vi "LC2_Comm_main.vi"() -> ()   [LabVIEW 2016]
uses:
  <vilib>/DNP3/DNP3_Master/Operation Mode.ctl
  <vilib>/DNP3/DNP3_Master/Poll Binary Input Variation.ctl
  <vilib>/DNP3/DNP3_Master/Analog Variation.ctl
  <vilib>/DNP3/DNP3_Master/Poll Analog Input Variation.ctl
  <vilib>/DNP3/DNP3_Master/Response Type.ctl
  <vilib>/DNP3/DNP3_Master/Start Stop.ctl
  <vilib>/DNP3/DNP3_Master/Analog Info.ctl
  BESS_LC/LC_BESS_global.vi
  Communication/Global communication.vi
  Communication/Global communication output.vi
  Communication/DNP3 communication files/MGCC Communication Files/DNP3_Master_Station_MGCC.lvlib
  <vilib>/DNP3/DNP3_Master.lvlib
panel:
  out "Startup time":dbl
  out "Array":T3(array[cluster])=[{"DNP3 channel"="Master/Channel 160.36.56.207: 18000", "DNP3 master"="Master", "DNP3 master session"="Master/Channel 160.36.56.207: 18000/Master Session 9-10", "DNP3 command"="Master/Channel 160.36.56.207: 18000/Master Session 9-10/Command ", "MS_Network_Settings_Initial"={"Outstation IP"="160.36.56.207", "DNP3 Port"=18000, "DNP3 Master Address"=9, "DNP3 Outstation Address"=10}, "Ping status"=enum."Success", "PollD"=[{"start"=0, "stop"=5}], "PollA"=[{"start"=0, "stop"=5}], "error out"={"status"=FALSE, "code"=5103, "source"="DNP3_Master_Station_MGCC.lvlib:LC1_MS_Main.vi:580001<ERR>\nCommunication timeout\n\n\n<b>Complete call chain:</b>\n     DNP3_Master_Station_MGCC.lvlib:LC1_MS_Main.vi:580001\n     LC2_Comm_main.vi"}, "MS_RESET_IND"=FALSE}]
  out "BESS LC communication":dbl[](array[numeric])=[0.0, 1.0369910801229782, 77.34308905073745, 0.0, 0.0, 0.5]
  out "OS SubVI Iterations":i16=6647
  in  "RESET OS":bool caption="Reset Outstation"
  in  "ENABLE OS":bool=TRUE
  out "OS SETTINGS CHANGED":bool
  out "MS POLLING? IND":bool=TRUE
  in  "Settings Cluster":T4={"Default Variation:Analog Input Event (OBJ32)"=1, "Default Variation:Analog Input (OBJ30)"=1, "Default Variation:Binary Input (OBJ01)"=1, "Default Variation:Analog Output (OBJ40)"=4, "Default Variation:Binary Output Event (OBJ11)"=1, "Default Variation:Binary Output (OBJ10)"=1, "Default Variation:Analog Output Event (OBJ42)"=8, "Unsolicited Response Allowed"=FALSE, "Control:Select Timeout (ms)"=0, "Misc:Appl Confirmation Timeout"=0} {"Default Variation:Analog Output Event (OBJ42)" items=["32-bit without Time"=1, "16-bit without Time"=2, "32-bit with Time"=3, "16-bit with Time"=4, "Single-prec without Time"=5, "Double-prec without Time"=6, "Single-prec with Time"=7, "Double-prec with Time"=8]; "Default Variation:Binary Output (OBJ10)" items=["Packed Format"=1, "Output Status with Flags"=2]; "Default Variation:Binary Output Event (OBJ11)" items=["Status without Time"=1, "Status with Time"=2]; "Default Variation:Analog Output (OBJ40)" items=["32-bit with Flag"=1, "16-bit with Flag"=2, "Single-prec with Flag"=3, "Double-prec with Flag"=4]; "Default Variation:Binary Input (OBJ01)" items=["Packed Format"=1, "With Flags"=2]; "Default Variation:Analog Input (OBJ30)" items=["32-bit with Flag"=1, "16-bit with Flag"=2, "32-bit without Flag"=3, "16-bit without Flag"=4, "Single-prec with Flag"=5, "Double-prec with Flag"=6]; "Default Variation:Analog Input Event (OBJ32)" items=["32-bit without Time"=1, "16-bit without Time"=2, "32-bit with Time"=3, "16-bit with Time"=4, "Single-prec without Time"=5, "Double-prec without Time"=6, "Single-prec with Time"=7, "Double-prec with Time"=8]}
  in  "Network Settings 1":T5={"port (20000)"=18000, "Master IP"="10.38.59.110", "Master Address"=12340, "Outstation Address "=54320, " update rate"=50}
  in  "DNP3 DataMap 1":T6={"Binary Output Points"=1, "Binary Input Points"=0, "Analog Output Points"=22, "Analog Input Points"=22}
  out "Numeric 3":i32
  out "LC1_MS_TX_Status_Binary":T1=enum."Cancel"
  out "LC1_MS_TX_Status_Analog":T1=enum."Success"
  out "LC1_MS_RX_Status_Binary":T1=enum."Cancel"
  out "LC1_MS_RX_Status_Analog":T1=enum."Success"
  out "Analog Input":dbl[](array[numeric])=[0.0, 1.0369911365960325, 77.34322413077294, 0.0, 0.0, 0.5]
  in  "LC1_MS_Network_Settings":T7={"Outstation IP"="160.36.56.207", "DNP3 Port"=18000, "DNP3 Master Address"=9, "DNP3 Outstation Address"=10}
  in  "Poll Enable":T8={"En_Rx_An"=TRUE, "En_Tx_An"=TRUE, "En_Rx_Di"=FALSE, "En_Tx_Di"=FALSE}
  in  "ENABLE MS":bool=TRUE
  in  "RESET MS":bool caption="Reset Outstation"
  in  "LC1_MS_DNP3_Settings":T13={"Binary Out Mode"=6, "Binary In Variation"=0, "Analog Out Variation"=4, "Analog Out Mode"=6, "Analog In Variation"=6} {"Analog In Variation" items=["Default", "32-bit with Flag", "16-bit with Flag", "32-bit without Flag", "16-bit without Flag", "Single-prec with Flag", "Double-prec with Flag"]; "Analog Out Mode" items=["SBO"=0, "Select"=3, "Operate"=4, "Direct"=5, "Direct No Ack"=6]; "Analog Out Variation" items=["32-bit"=1, "16-bit"=2, "Single-prec"=3, "Double-prec"=4]; "Binary In Variation" items=["Default", "Packed Format", "With Flags"]; "Binary Out Mode" items=["SBO"=0, "Select"=3, "Operate"=4, "Direct"=5, "Direct No Ack"=6]}
  out "Numeric":i32=3331
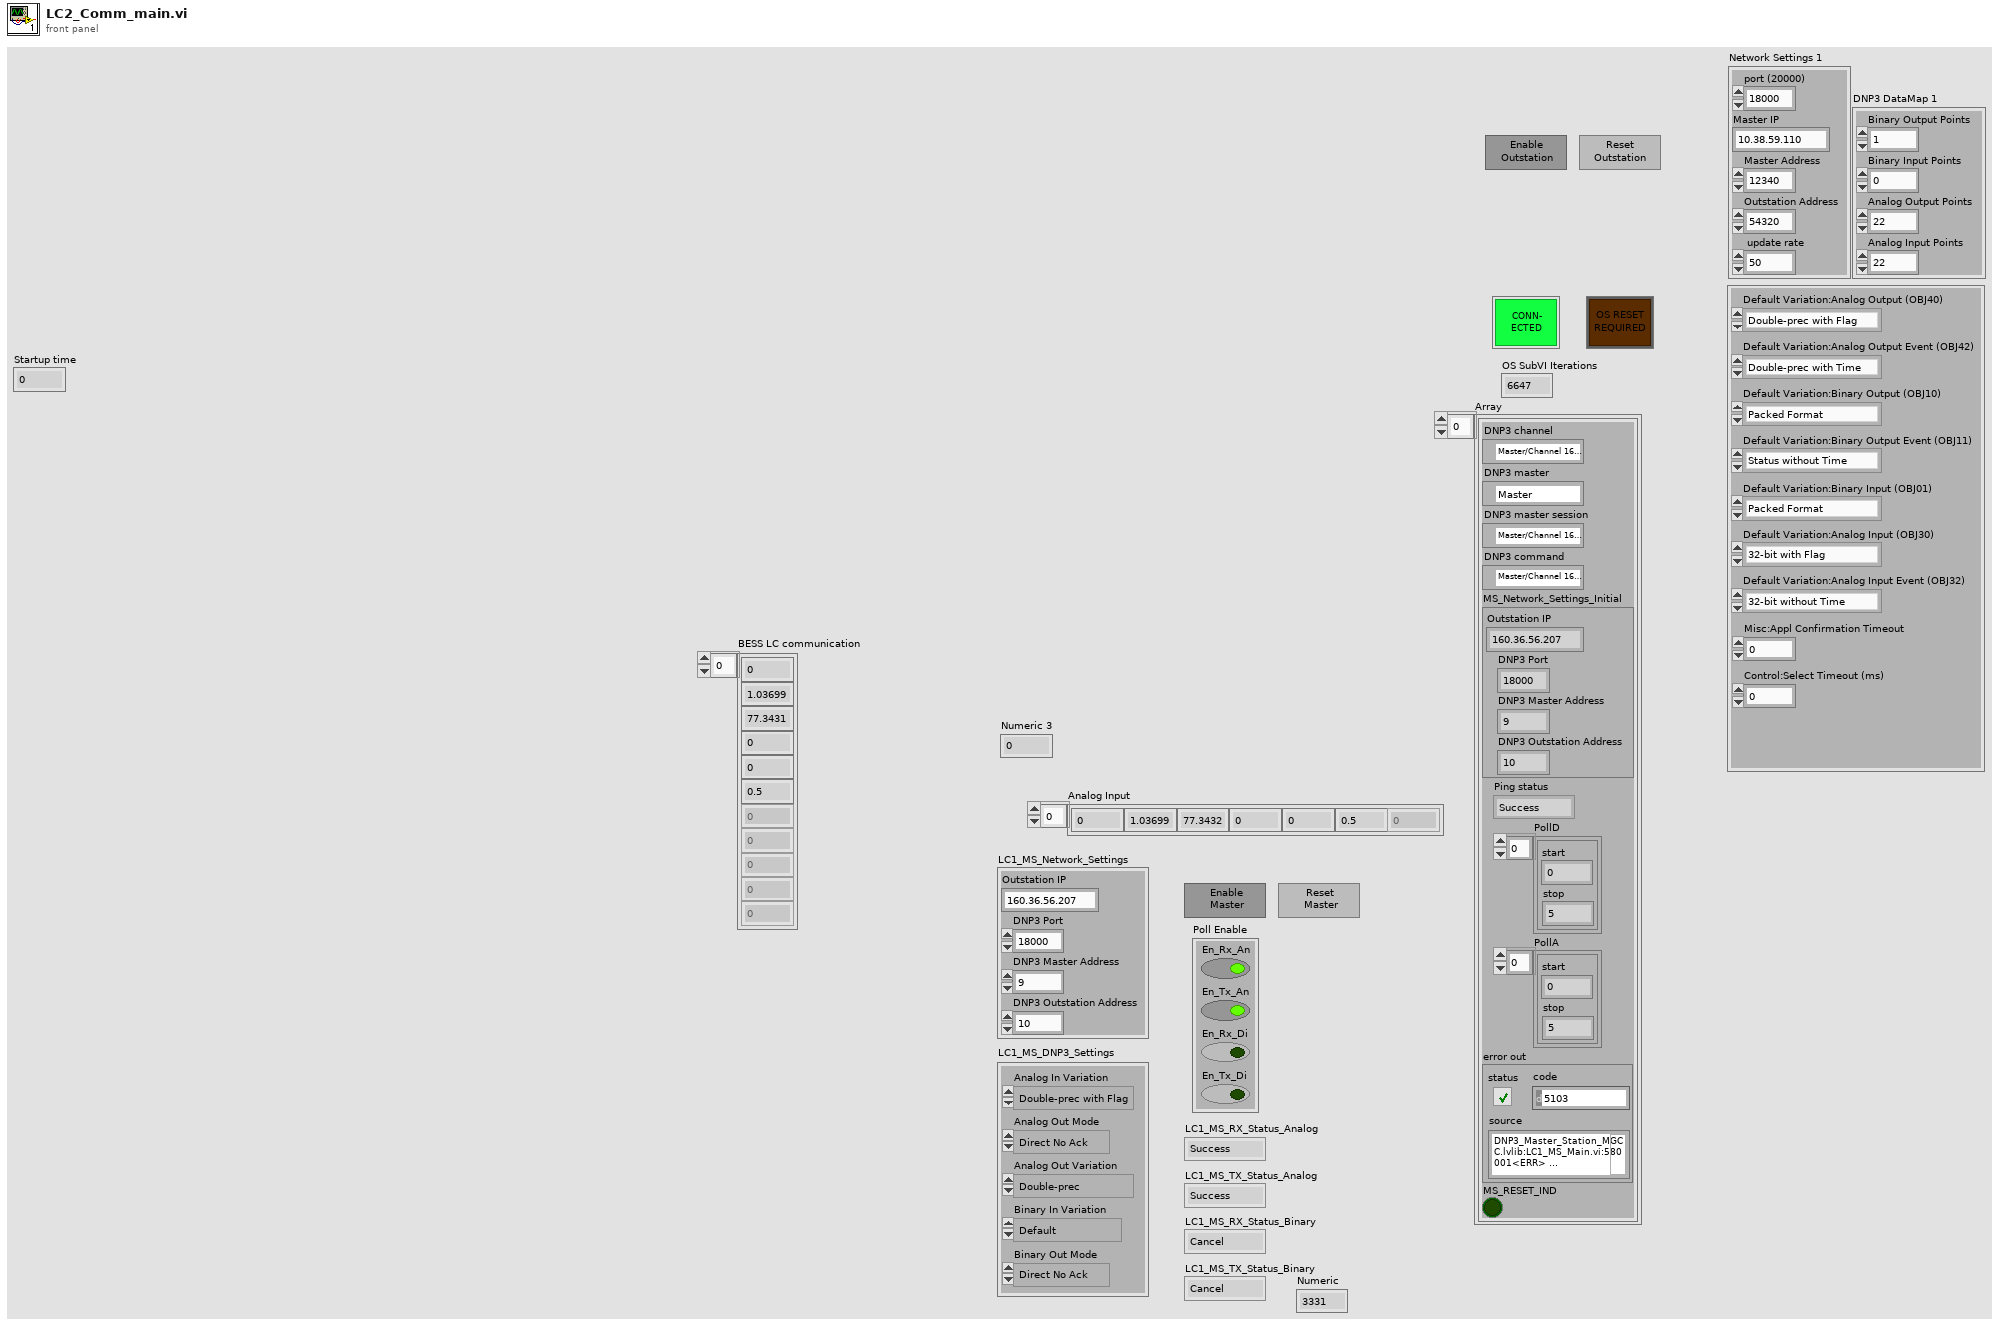
[diagram p1: front panel]
types:
  T1 = typedef "DNP3_Master.lvlib/Response Type.ctl" = enum16{"Idle", "Buffering", "Pending", "Success", "Failure", "Mismatch", "Status Code", "IIN", "Timeout", "Cancel"}
  T2 = typedef "DNP3_Master.lvlib/Start Stop.ctl" = cluster{"start":u16, "stop":u16}
  T3 = cluster{"DNP3 channel":refnum<k21>, "DNP3 master":refnum<k21>, "DNP3 master session":refnum<k21>, "DNP3 command":refnum<k21>, "MS_Network_Settings_Initial":cluster{"Outstation IP":string, "DNP3 Port":u16, "DNP3 Master Address":u16, "DNP3 Outstation Address":u16}, "Ping status":T1, "PollD":T2[], "PollA":T2[], "error out":errorcluster, "MS_RESET_IND":bool}[]
  T4 = cluster{"Default Variation:Analog Input Event (OBJ32)":u8, "Default Variation:Analog Input (OBJ30)":u8, "Default Variation:Binary Input (OBJ01)":u8, "Default Variation:Analog Output (OBJ40)":u8, "Default Variation:Binary Output Event (OBJ11)":u8, "Default Variation:Binary Output (OBJ10)":u8, "Default Variation:Analog Output Event (OBJ42)":u8, "Unsolicited Response Allowed":bool, "Control:Select Timeout (ms)":u32, "Misc:Appl Confirmation Timeout":u32}
  T5 = cluster{"port (20000)":u16, "Master IP":string, "Master Address":u16, "Outstation Address ":u16, " update rate":u32}
  T6 = cluster{"Binary Output Points":u16, "Binary Input Points":u16, "Analog Output Points":u16, "Analog Input Points":u16}
  T7 = cluster{"Outstation IP":string, "DNP3 Port":u16, "DNP3 Master Address":u16, "DNP3 Outstation Address":u16}
  T8 = cluster{"En_Rx_An":bool, "En_Tx_An":bool, "En_Rx_Di":bool, "En_Tx_Di":bool}
  T9 = typedef "DNP3_Master.lvlib/Operation Mode.ctl" = u8
  T10 = typedef "DNP3_Master.lvlib/Poll Binary Input Variation.ctl" = u8
  T11 = typedef "DNP3_Master.lvlib/Analog Variation.ctl" = u8
  T12 = typedef "DNP3_Master.lvlib/Poll Analog Input Variation.ctl" = u8
  T13 = cluster{"Binary Out Mode":T9, "Binary In Variation":T10, "Analog Out Variation":T11, "Analog Out Mode":T9, "Analog In Variation":T12}
  T14 = typedef "DNP3_Master.lvlib/Analog Info.ctl" = cluster{"index":u16, "value":dbl}
  T15 = cluster{"Binary Out Mode":T9, "Binary In Variation":T10, "Analog Out Variation":T11, "Analog Out Mode":T9, "Analog In Variation":T12}[]
  T16 = cluster{"En_Rx_An":bool, "En_Tx_An":bool, "En_Rx_Di":bool, "En_Tx_Di":bool}[]
  T17 = cluster{"Outstation IP":string, "DNP3 Port":u16, "DNP3 Master Address":u16, "DNP3 Outstation Address":u16}[]
  T18 = cluster{"response status":T1, "response status":T1, "response status":T1, "response status":T1}
  T19 = cluster{"DNP3 channel":refnum<k21>, "DNP3 master":refnum<k21>, "DNP3 master session":refnum<k21>, "DNP3 command":refnum<k21>, "MS_Network_Settings_Initial":cluster{"Outstation IP":string, "DNP3 Port":u16, "DNP3 Master Address":u16, "DNP3 Outstation Address":u16}, "Ping status":T1, "PollD":T2[], "PollA":T2[], "error out":errorcluster, "MS_RESET_IND":bool}
  T20 = cluster{"DNP3 outstation session out":refnum<k21>, "DNP3 outstation out":refnum<k21>, "error out":errorcluster}
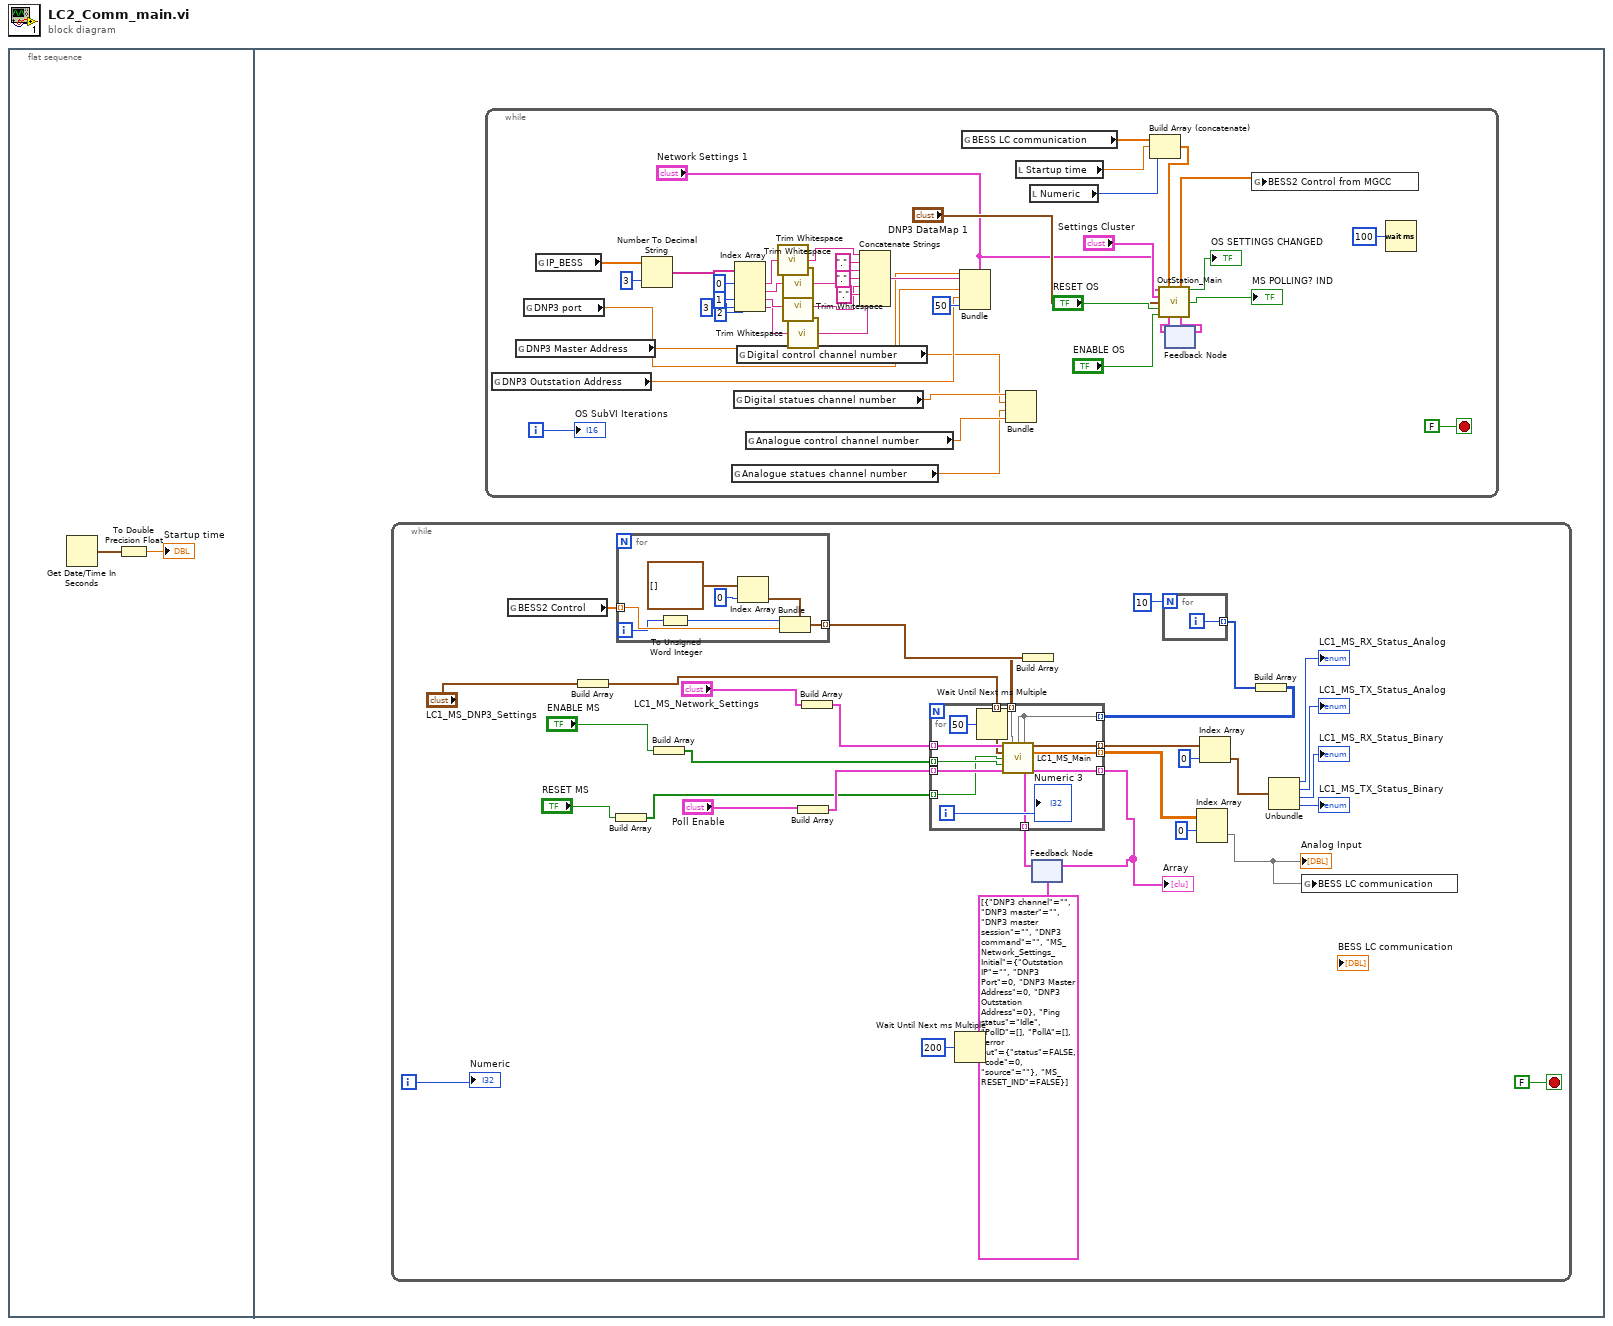
[diagram p0: block diagram]
diagram:
  n1 = flat-sequence {
    frame #0 {
      n2 = Get Date/Time In Seconds() -> (seconds since 1Jan1904=w2:timestamp)
      n3 = To Double Precision Float(number=w2) -> (double precision float=→"Startup time":dbl)
    }
    frame #1 {
      n4 = while {
        i -> [w9]
        stop <- FALSE stop-if-true
        n5 = global read "Global communication output.vi" "BESS2 Control"() -> (w13:dbl[])
        n6 = Build Array("LC1_MS_DNP3_Settings") -> (w14:T15)
        n7 = Build Array("RESET MS") -> (w16:bool[])
        n8 = for {
          tunnel: [w42] -> w12 mode=indexing
          tunnel: w13 -> [w37] mode=indexing
          i -> [w36]
          n9 = To Unsigned Word Integer(number=w36) -> (unsigned 16bit integer=w38:u16)
          n10 = Index Array(array=T14[] [] ("values"), index=0) -> (element=w39:T14)
          n11 = Bundle(cluster=w39, "index"=w38, "value"=w37) -> (w42:T14)
        }
        n12 = Build Array("ENABLE MS") -> (w18:bool[])
        n13 = Build Array("Poll Enable") -> (w20:T16)
        n14 = Build Array("LC1_MS_Network_Settings") -> (w22:T17)
        n15 = Wait Until Next ms Multiple(millisecond multiple=u32 200) -> ()  [unwired: 1 out]
        n16 = Build Array(w12) -> (w11:T14[][])
        n17 = feedback #1(T3 [{"DNP3 channel"="", "DNP3 master"="", "DNP3 master session"="", "DNP3 command"="", "MS_Network_Settings_Initial"={"Outstation IP"="", "DNP3 Port"=0, "DNP3 Master Address"=0, "DNP3 Outstation Address"=0}, "Ping status"=enum."Idle", "PollD"=[], "PollA"=[], "error out"={"status"=FALSE, "code"=0, "source"=""}, "MS_RESET_IND"=FALSE}]) -> (w6:T3)
        n18 = for {
          N: 10 -> [_]
          tunnel: [w35] -> w3 mode=indexing
          i -> [w35]
        }
        n19 = Build Array(w3) -> (w10:i32[][])
        n20 = for {
          tunnel: [w55] -> w30 mode=indexing
          tunnel: [w54] -> w25 mode=indexing
          tunnel: w22 -> [w53] mode=indexing
          tunnel: [w52] -> w7 mode=indexing
          tunnel: w20 -> [w51] mode=indexing
          tunnel: w18 -> [w50] mode=indexing
          tunnel: w16 -> [w49] mode=indexing
          tunnel: w14 -> [w48] mode=indexing
          tunnel: w11 -> [w47] mode=indexing
          tunnel: w10 -> [w46] mode=indexing
          tunnel: w6 -> [w43] mode=indexing
          i -> [w45]
          n21 = Wait Until Next ms Multiple(millisecond multiple=u32 50) -> ()  [unwired: 1 out]
          n22 = call "LC1_MS_Main.vi"("MS_Network_Settings"=w53, "Analog Output"=w47, "Analog Input Indexes"=w46, "Digital Input Indexes"=w46, "MS_DNP3_Settings"=w48, "MS_RESET"=w49, "MS_ENABLE"=w50, "Poll Enable"=w51, "DNP3 Session Feedback"=w43) -> ("Comm Status"=w55:T18, "Analog Input"=w54:dbl[], "DNP3 Session Output"=w52:T19)  [unwired: 3 in, 1 out]
          "Numeric 3" <- w45
        }
        "Array" <- w7
        n23 = feedback-in #1(w7) -> ()
        n24 = Index Array(array=w25, index (row)=0 ("index")) -> (element=w26:dbl[])  [unwired: 1 in]
        "Analog Input" <- w26
        n25 = Index Array(array=w30, index=0) -> (element=w29:T18)
        n26 = Unbundle(w29) -> ("response status"=→"LC1_MS_RX_Status_Analog":T1, "response status"=→"LC1_MS_TX_Status_Analog":T1, "response status"=→"LC1_MS_RX_Status_Binary":T1, "response status"=→"LC1_MS_TX_Status_Binary":T1)
        n27 = global write "Global communication.vi" "BESS LC communication"(w26) -> ()
        "Numeric" <- w9
      }
      n28 = while {
        i -> [w97]
        stop <- FALSE stop-if-true
        n29 = global read "LC_BESS_global.vi" "DNP3 Outstation Address"() -> (w74:dbl)
        n30 = global read "LC_BESS_global.vi" "DNP3 Master Address"() -> (w75:dbl)
        n31 = global read "LC_BESS_global.vi" "DNP3 port"() -> (w76:dbl)
        n32 = global read "LC_BESS_global.vi" "IP_BESS"() -> (w95:dbl[])
        n33 = Number To Decimal String(number=w95, width (-)=i16 3) -> (decimal integer string=w93:string[])
        n34 = global read "LC_BESS_global.vi" "Analogue statues channel number"() -> (w70:dbl)
        n35 = global read "LC_BESS_global.vi" "Digital statues channel number"() -> (w73:dbl)
        n36 = Index Array(array=w93, index #1=0 ("index"), index #2=1 ("index"), index #3=2 ("index"), index #4=3 ("index")) -> (element #1=w85:string, element #2=w83:string, element #3=w81:string, element #4=w79:string)
        n37 = global read "LC_BESS_global.vi" "Digital control channel number"() -> (w72:dbl)
        n38 = global read "LC_BESS_global.vi" "Analogue control channel number"() -> (w71:dbl)
        n39 = call <vilib>:"Trim Whitespace.vi"("string"=w85) -> ("trimmed string"=w84:string)  [unwired: 1 in]
        n40 = call <vilib>:"Trim Whitespace.vi"("string"=w83) -> ("trimmed string"=w82:string)  [unwired: 1 in]
        n41 = call <vilib>:"Trim Whitespace.vi"("string"=w81) -> ("trimmed string"=w80:string)  [unwired: 1 in]
        n42 = call <vilib>:"Trim Whitespace.vi"("string"=w79) -> ("trimmed string"=w78:string)  [unwired: 1 in]
        n43 = Concatenate Strings(w84, "." ("string"), w82, "." ("string"), w80, "." ("string"), w78) -> (w77:string)
        n44 = Bundle(cluster="Network Settings 1", "port (20000)"=w76, "Master IP"=w77, "Master Address"=w75, "Outstation Address"=w74, "update rate"=u32 50) -> ()  [unwired: 1 out]
        n45 = global read "Global communication.vi" "BESS LC communication"() -> (w59:dbl[])
        n46 = Bundle("Digital statues channel number"=w73, "Digital control channel number"=w72, "Analogue statues channel number"=w70, "Analogue control channel number"=w71) -> ()  [unwired: 1 in, 1 out]
        n47 = local read "Startup time"() -> (w58:dbl)
        n48 = local read "Numeric"() -> (w57:i32)
        n49 = Build Array (concatenate)(w59, w58, w57) -> (w56:dbl[])
        n50 = feedback #2() -> (w65:T20)  [unwired: 1 in]
        n51 = call "OutStation_Main.vi"("Network Settings 1"="Network Settings 1", "Analog Input"=w56, "Settings Cluster"="Settings Cluster", "DNP3 DataMap 1"="DNP3 DataMap 1", "OS_Reset"="RESET OS", "OS_Enable"="ENABLE OS", "DNP3 Session Input"=w65) -> ("Analog Output"=w60:dbl[], "OS_DNP3_Settings_Changed"=→"OS SETTINGS CHANGED":bool, "Connected?"=→"MS POLLING? IND":bool, "DNP3 Session"=w66:T20)  [unwired: 2 in, 3 out]
        n52 = feedback-in #2(w66) -> ()
        n53 = global write "Global communication output.vi" "BESS2 Control from MGCC"(w60) -> ()
        n54 = Wait (ms)(milliseconds to wait=u32 100) -> ()  [unwired: 1 out]
        "OS SubVI Iterations" <- w97
      }
    }
  }
